vi "macro_AutoHelp_Sequence.vi"   [LabVIEW 2019, in "Trajectory_Library.lvlib"]
uses:
  Trajectory_Library.lvlib
types:
  T1 = typedef "Trajectory_Library.lvlib/AutoHelperSequence_Step_Enum.ctl" = enum16{"WaitingForAutoToStart", "Step 1", "Step 2", "Step 3", "Step 4", "Step 5", "Step 6", "Step 7", "Step 8", "Step 9", "Step 10", "Step 11", "Step 12", "Step 13", "Step 14", "Step 15", "Step 16", "Step 17", "Step 18", "Step 19", "Step 20", "Step 21", "Step 22", "Step 23", "Step 24", "Step 25", "Step 26", "Step 27", "Step 28", "Step 29", "Step 30", "Step 31", "Step 32", "AutoDone"}
  T2 = typedef "Trajectory_Library.lvlib/CHASSIS_SPEEDS.ctl" = cluster{"vX":dbl, "vY":dbl, "vOmega":dbl}
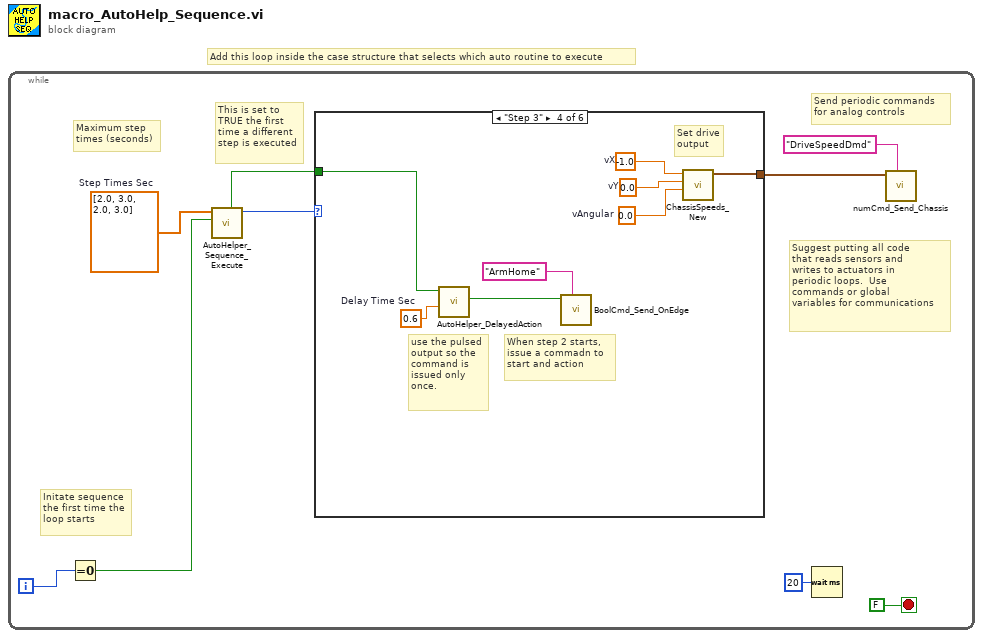
[diagram p0: block diagram]
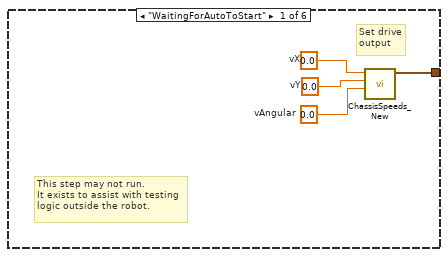
[diagram p2: hidden frame]
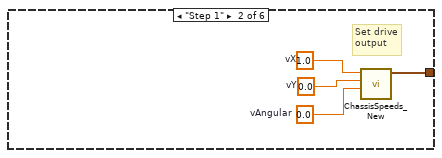
[diagram p3: hidden frame]
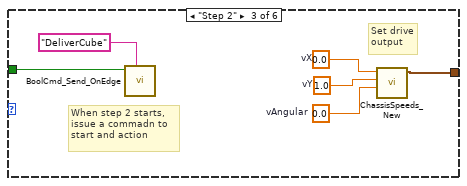
[diagram p4: hidden frame]
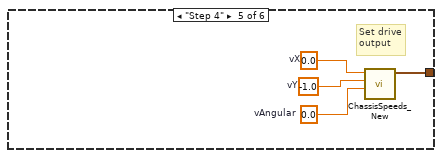
[diagram p5: hidden frame]
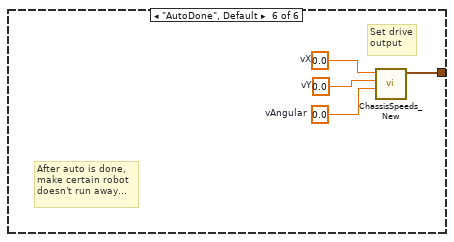
[diagram p6: hidden frame]
diagram:
  # "Add this loop inside the case structure that selects which auto routine to execute"
  n1 = while {
    i -> [w7]
    stop <- FALSE stop-if-true
    w5 = dbl[] [2.0, 3.0, 2.0, 3.0]  # Step Times Sec
    # "Suggest putting all code\nthat reads sensors and\nwrites to actuators in\nperiodic loops.  Use\ncommands or global\nvariables for communications"
    # "Send periodic commands\nfor analog controls"
    # "This is set to\nTRUE the first\ntime a different\nstep is executed"
    # "Maximum step\ntimes (seconds)"
    # "Initate sequence\nthe first time the\nloop starts"
    n2 = Equal To 0?(x=w7) -> (x = 0?=w6:bool)
    n3 = call "AutoHelper_Sequence_Execute.vi"("Initiate"=w6, "Step Times Sec"=w5) -> ("Step Number State"=w3:T1, "New Step"=w4:bool)  [unwired: 5 in, 3 out]
    n4 = case shown="\"Step 3\"" w3 {
      tunnel: w4 -> [_ _ w19 w24 _ _]
      tunnel: [w10 w14 w20 w28 w32 w36] -> w1
      frame "WaitingForAutoToStart" {
        w11 = 0.0  # vX
        w12 = 0.0  # vY
        w13 = 0.0  # vAngular
        # "Set drive\noutput"
        # "This step may not run.  \nIt exists to assist with testing\nlogic outside the robot."
        n5 = call "ChassisSpeeds_New.vi"("vAngular"=w13, "vY"=w12, "vX"=w11) -> ("CHASSIS"=w10:T2)  [unwired: 8 in]
      }
      frame "Step 1" {
        w15 = 1.0  # vX
        w16 = 0.0  # vY
        w17 = 0.0  # vAngular
        # "Set drive\noutput"
        n6 = call "ChassisSpeeds_New.vi"("vAngular"=w17, "vY"=w16, "vX"=w15) -> ("CHASSIS"=w14:T2)  [unwired: 8 in]
      }
      frame "Step 2" {
        w21 = 0.0  # vX
        w22 = 1.0  # vY
        w23 = 0.0  # vAngular
        # "When step 2 starts, \nissue a commadn to\nstart and action"
        # "Set drive\noutput"
        n7 = call "BoolCmd_Send_OnEdge.vi"("Command Name"="DeliverCube", "Value"=w19) -> ()  [unwired: 9 in, 1 out]
        n8 = call "ChassisSpeeds_New.vi"("vAngular"=w23, "vY"=w22, "vX"=w21) -> ("CHASSIS"=w20:T2)  [unwired: 8 in]
      }
      frame "Step 3" {
        w25 = 0.6  # Delay Time Sec
        w29 = -1.0  # vX
        w30 = 0.0  # vY
        w31 = 0.0  # vAngular
        # "use the pulsed\noutput so the\ncommand is\nissued only\nonce."
        # "When step 2 starts, \nissue a commadn to\nstart and action"
        # "Set drive\noutput"
        n9 = call "AutoHelper_DelayedAction.vi"("Delay Time Sec"=w25, "New Step"=w24) -> ("Delayed Action Pulse"=w26:bool)  [unwired: 5 in, 4 out]
        n10 = call "BoolCmd_Send_OnEdge.vi"("Command Name"="ArmHome", "Value"=w26) -> ()  [unwired: 9 in, 1 out]
        n11 = call "ChassisSpeeds_New.vi"("vAngular"=w31, "vY"=w30, "vX"=w29) -> ("CHASSIS"=w28:T2)  [unwired: 8 in]
      }
      frame "Step 4" {
        w33 = 0.0  # vX
        w34 = -1.0  # vY
        w35 = 0.0  # vAngular
        # "Set drive\noutput"
        n12 = call "ChassisSpeeds_New.vi"("vAngular"=w35, "vY"=w34, "vX"=w33) -> ("CHASSIS"=w32:T2)  [unwired: 8 in]
      }
      frame "AutoDone", Default {
        w37 = 0.0  # vX
        w38 = 0.0  # vY
        w39 = 0.0  # vAngular
        # "After auto is done,\nmake certain robot\ndoesn't run away..."
        # "Set drive\noutput"
        n13 = call "ChassisSpeeds_New.vi"("vAngular"=w39, "vY"=w38, "vX"=w37) -> ("CHASSIS"=w36:T2)  [unwired: 8 in]
      }
    }
    n14 = Wait (ms)(milliseconds to wait=u32 20) -> ()  [unwired: 1 out]
    n15 = call "numCmd_Send_Chassis.vi"("Command Name"="DriveSpeedDmd", "Chassis Speeds"=w1) -> ()  [unwired: 9 in, 1 out]
  }
